vi "Configure Trigger Settings Dialog.vi"(8 "error in":errorcluster, 11 "Script Trigger Settings Ref":refnum<vi>) -> (0 "error out":errorcluster)   [LabVIEW 2025, in "Fgen Script Mode UI.lvlib"]
uses:
  Fgen Script Mode UI.lvlib
  <vilib>/ErrorRing/Error Ring.xnode
  Typedef/Trigger Settings.ctl
panel:
  in  "Tab Control":enum32{"Script Triggers", "Markers"}(tab)
  in  "Script Trigger 0 Source":tag
  in  "Script Trigger 1 Source":tag
  in  "Script Trigger 2 Source":tag
  in  "Script Trigger 3 Source":tag
  in  "Marker3 Output Terminal":string(combo)
  in  "Marker2 Output Terminal":string(combo)
  in  "Marker1 Output Terminal":string(combo)
  in  "Marker0 Output Terminal":string(combo)
  in  "Cancel":bool
  in  "OK":bool
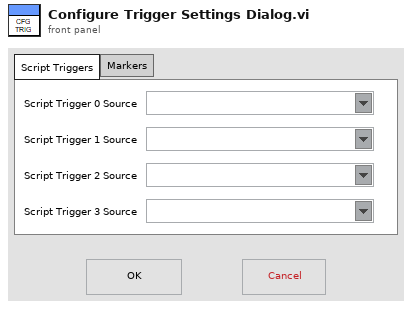
[diagram p1: front panel]
types:
  T1 = typedef "Fgen Script Mode UI.lvlib/Trigger Settings.ctl" = cluster{"Script Trigger 0 Source":string, "Script Trigger 1 Source":string, "Script Trigger 2 Source":string, "Script Trigger 3 Source":string, "Marker0 Output Terminal":string, "Marker1 Output Terminal":string, "Marker2 Output Terminal":string, "Marker3 Output Terminal":string}
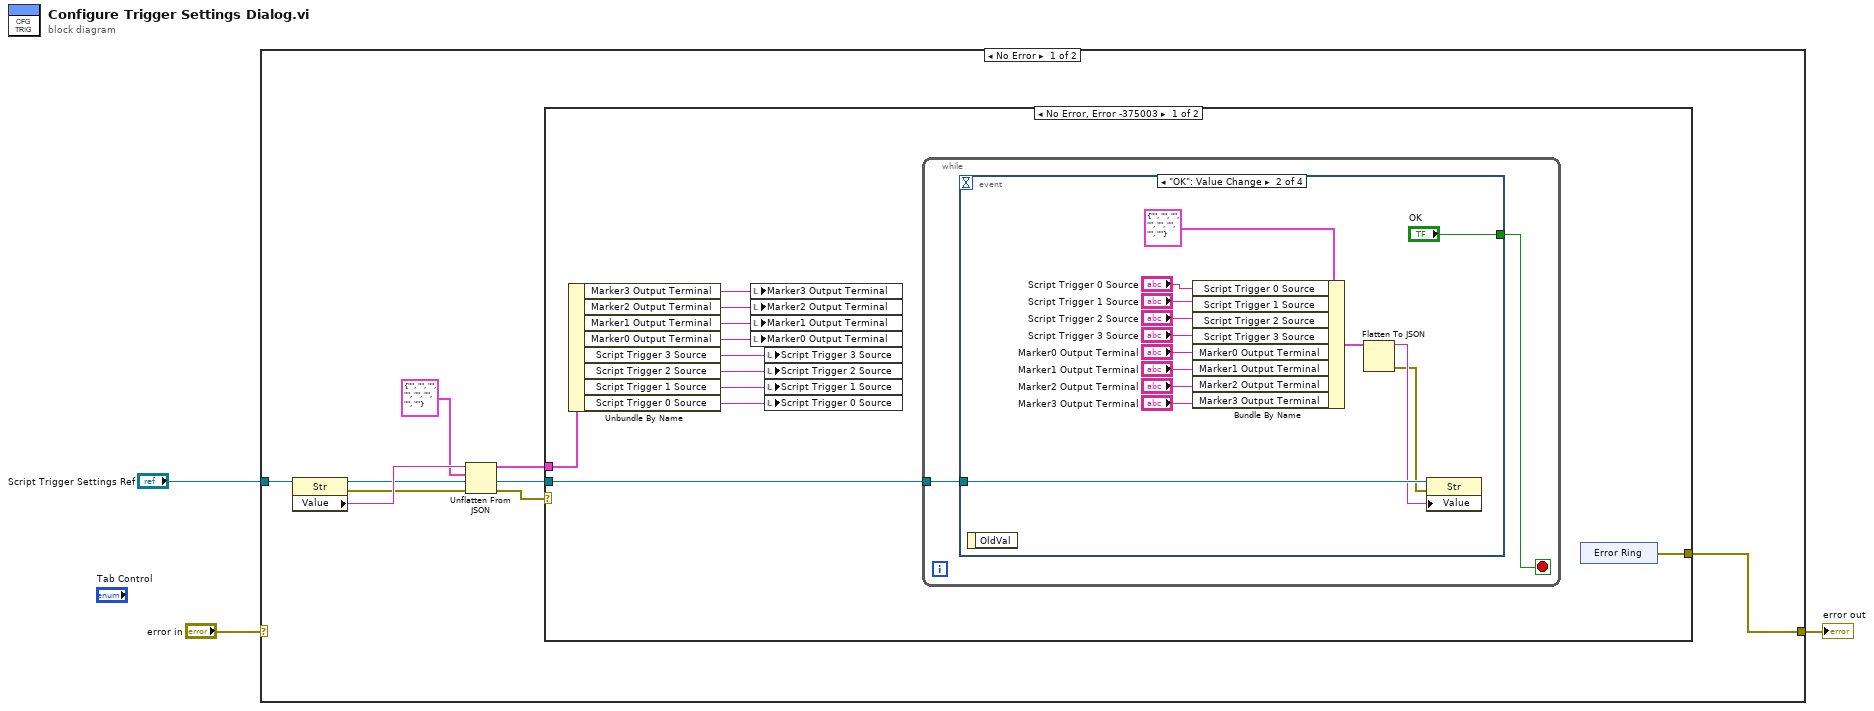
[diagram p0: block diagram]
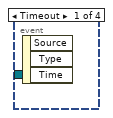
[diagram p2: hidden frame]
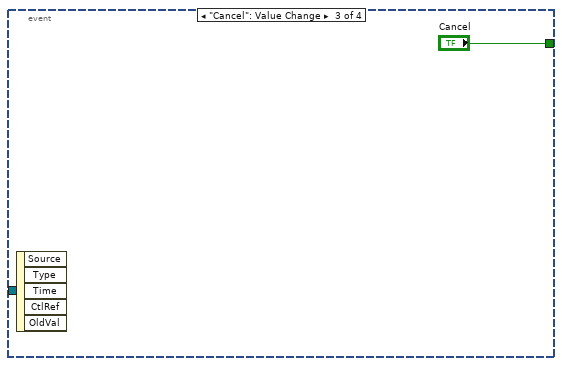
[diagram p3: hidden frame]
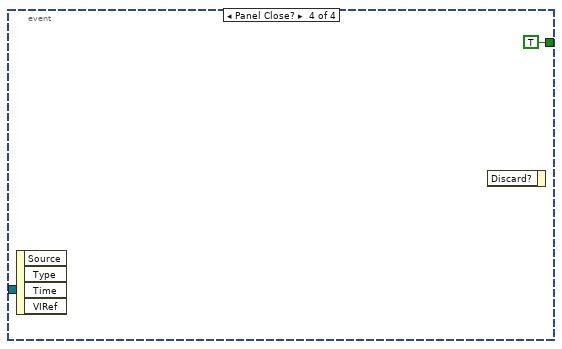
[diagram p4: hidden frame]
diagram:
  n1 = case shown="No Error" "error in" {
    selector: "error in" -> [_ w43]
    tunnel: [w5 w43] -> w2
    tunnel: "Script Trigger Settings Ref" -> [w11 _]
    frame No Error {
      n2 = property class="Str"(reference=w11) -> (reference out=w6:refnum<vi>, error out=w9:errorcluster, "Value"=w10:string)  [unwired: 1 in]
      n3 = Unflatten From JSON(JSON string=w10, type and defaults=T1 {"Script Trigger 0 Source"="", "Script Trigger 1 Source"="", "Script Trigger 2 Source"="", "Script Trigger 3 Source"="", "Marker0 Output Terminal"="", "Marker1 Output Terminal"="", "Marker2 Output Terminal"="", "Marker3 Output Terminal"=""} ("Trigger Settings"), error in (no error)=w9) -> (value=w7:T1, error out=w8:errorcluster)  [unwired: 4 in]
      n4 = case shown="No Error, Error -375003" w8 {
        selector: w8 -> [_ w42]
        tunnel: w7 -> [w21 _]
        tunnel: [w22 w42] -> w5
        tunnel: w6 -> [w12 _]
        frame No Error {
          n5 = Unbundle By Name(w21) -> ("Marker3 Output Terminal"=w13:string, "Marker2 Output Terminal"=w14:string, "Marker1 Output Terminal"=w15:string, "Marker0 Output Terminal"=w16:string, "Script Trigger 3 Source"=w17:string, "Script Trigger 2 Source"=w18:string, "Script Trigger 1 Source"=w19:string, "Script Trigger 0 Source"=w20:string)
          n6 = local write "Marker3 Output Terminal"(w13) -> ()
          n7 = local write "Marker2 Output Terminal"(w14) -> ()
          n8 = local write "Marker1 Output Terminal"(w15) -> ()
          n9 = local write "Marker0 Output Terminal"(w16) -> ()
          n10 = local write "Script Trigger 3 Source"(w17) -> ()
          n11 = local write "Script Trigger 2 Source"(w18) -> ()
          n12 = local write "Script Trigger 1 Source"(w19) -> ()
          n13 = local write "Script Trigger 0 Source"(w20) -> ()
          n14 = while {
            tunnel: w12 -> [w23]
            stop <- w24 stop-if-true
            n15 = event shown="[1] \"OK\": Value Change" {
              selector: _ -> [_ _ _ _]
              dyn-events: _ -> [_ _ _ _]
              timeout: _ -> [_ _ _ _]
              tunnel: [_ "OK" "Cancel" TRUE ("Cancel")] -> w24
              tunnel: w23 -> [_ w27 _ _]
              event Timeout {
                n16 = event-data() -> ()  [unwired: 1 in, 3 out]
              }
              event "OK": Value Change {
                n17 = event-data() -> ()  [unwired: 1 in, 1 out]
                n18 = Bundle By Name(cluster=T1 {"Script Trigger 0 Source"="", "Script Trigger 1 Source"="", "Script Trigger 2 Source"="", "Script Trigger 3 Source"="", "Marker0 Output Terminal"="", "Marker1 Output Terminal"="", "Marker2 Output Terminal"="", "Marker3 Output Terminal"=""} ("Trigger Settings"), "Script Trigger 0 Source"="Script Trigger 0 Source", "Script Trigger 1 Source"="Script Trigger 1 Source", "Script Trigger 2 Source"="Script Trigger 2 Source", "Script Trigger 3 Source"="Script Trigger 3 Source", "Marker0 Output Terminal"="Marker0 Output Terminal", "Marker1 Output Terminal"="Marker1 Output Terminal", "Marker2 Output Terminal"="Marker2 Output Terminal", "Marker3 Output Terminal"="Marker3 Output Terminal") -> (w28:T1)
                n19 = Flatten To JSON(anything=w28) -> (JSON string=w26:string, 11:w25:errorcluster)  [unwired: 2 in]
                n20 = property class="Str"(reference=w27, error in=w25, "Value"=w26) -> ()  [unwired: 2 out]
              }
              event "Cancel": Value Change {
                n21 = event-data() -> ()  [unwired: 1 in, 5 out]
              }
              event Panel Close? {
                n22 = event-data() -> ()  [unwired: 1 in, 4 out]
                n23 = event-data() -> ()  [unwired: 2 in, 1 out]
              }
            }
          }
          n24 = xnode "Error Ring"() -> ("error out"=w22:errorcluster)
        }
        frame Default {
        }
      }
    }
    frame Error {
    }
  }
  "error out" <- w2
